vi "Test for OOB Services.vi"(8 "error in":errorcluster, 11 "address":string) -> (0 "error out":errorcluster, 3 "Found OOB Server":bool)   [LabVIEW 2026]
uses:
  Ref/reflection_client/RPC Messages/grpc_reflection_v1alpha_ServiceResponse.ctl
  Ref/reflection_client/RPC Messages/grpc_reflection_v1alpha_ServerReflectionRequest.ctl
  Ref/reflection_client/RPC Messages/grpc_reflection_v1alpha_ServerReflectionRequest_message_request/grpc_reflection_v1alpha_ServerReflectionRequest_message_request.lvclass
  Ref/reflection_client/RPC Messages/grpc_reflection_v1alpha_ServerReflectionRequest_message_request/grpc_reflection_v1alpha_ServerReflectionRequest_message_request.lvclass/grpc_reflection_v1alpha_ServerReflectionRequest_message_request.ctl
  Ref/reflection_client/RPC Messages/grpc_reflection_v1alpha_ServerReflectionResponse_message_response/grpc_reflection_v1alpha_ServerReflectionResponse_message_response.lvclass/grpc_reflection_v1alpha_ServerReflectionResponse_message_response.ctl
  Ref/reflection_client.lvlib
  Ref/reflection_client/RPC Messages/grpc_reflection_v1alpha_ServerReflectionResponse_message_response/grpc_reflection_v1alpha_ServerReflectionResponse_message_response.lvclass
panel:
  out "service":T1[](array[typedef])
  out "Success":bool
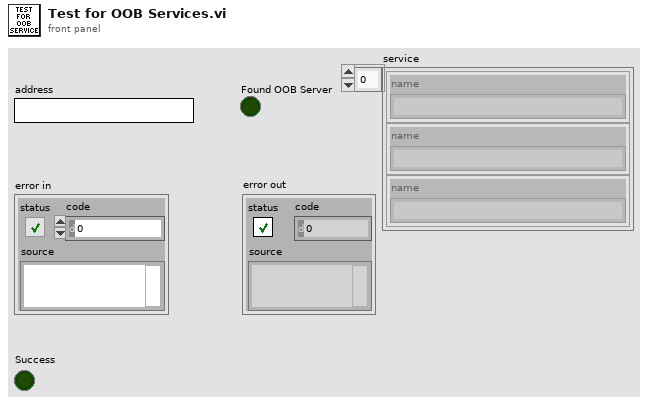
[diagram p1: front panel]
types:
  T1 = typedef "reflection_client.lvlib/grpc_reflection_v1alpha_ServiceResponse.ctl" = cluster{"name":string}
  T2 = typedef "reflection_client.lvlib/grpc_reflection_v1alpha_ServerReflectionRequest.ctl" = cluster{"host":string, "grpc_reflection_v1alpha_ServerReflectionRequest_message_request":refnum<class "grpc_reflection_v1alpha_ServerReflectionRequest_message_request.lvclass">}
  T3 = typedef "grpc-lvsupport-release.lvlib/grpcId.ctl" = u64
  T4 = typedef "reflection_client.lvlib/grpc_reflection_v1alpha_ServerReflectionResponse.ctl" = cluster{"valid_host":string, "original_request":T2, "grpc_reflection_v1alpha_ServerReflectionResponse_message_response":refnum<class "grpc_reflection_v1alpha_ServerReflectionResponse_message_response.lvclass">}
  T5 = typedef "reflection_client.lvlib/grpc_reflection_v1alpha_ListServiceResponse.ctl" = cluster{"service":T1[]}
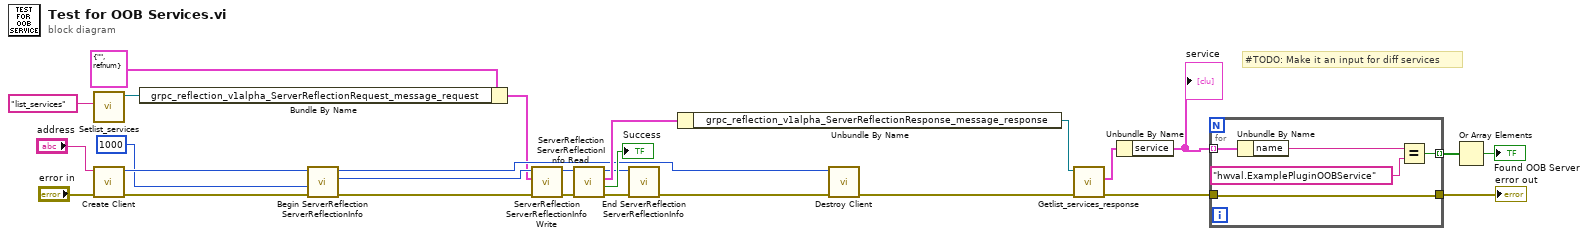
[diagram p0: block diagram]
diagram:
  # "#TODO: Make it an input for diff services"
  n1 = call "Setlist_services.vi"("Set_Val"="list_services") -> ("OneOfTemplate out"=w14:refnum<class "grpc_reflection_v1alpha_ServerReflectionRequest_message_request.lvclass">)  [unwired: 9 in, 1 out]
  n2 = call "Create Client.vi"("error in"="error in", "address"="address") -> ("error out"=w24:errorcluster, "gRPC ID Out"=w25:T3)  [unwired: 8 in]
  n3 = Bundle By Name(cluster=T2 {"host"="", "grpc_reflection_v1alpha_ServerReflectionRequest_message_request"=refnum} ("Request Data"), "grpc_reflection_v1alpha_ServerReflectionRequest_message_request"=w14) -> (w10:T2)
  n4 = call "Begin ServerReflection ServerReflectionInfo.vi"("error in"=w24, "timeout (ms)"=1000, "gRPC ID"=w25) -> ("error out"=w17:errorcluster, "Call Id Out"=w18:T3, "gRPC ID out"=w12:T3)  [unwired: 6 in]
  n5 = call "ServerReflection ServerReflectionInfo Write.vi"("error in"=w17, "Request Data"=w10, "Call ID in"=w18) -> ("error out"=w15:errorcluster, "Call ID"=w16:T3)  [unwired: 6 in, 1 out]
  n6 = call "ServerReflection ServerReflectionInfo Read.vi"("error in"=w15, "Call ID in"=w16) -> ("error out"=w9:errorcluster, "Success"=→"Success":bool, "Response Data"=w21:T4, "Call ID"=w7:T3)  [unwired: 6 in]
  n7 = call "End ServerReflection ServerReflectionInfo.vi"("error in"=w9, "Call ID in"=w7) -> ("error out"=w8:errorcluster)  [unwired: 8 in, 1 out]
  n8 = Unbundle By Name(w21) -> ("grpc_reflection_v1alpha_ServerReflectionResponse_message_response"=w20:refnum<class "grpc_reflection_v1alpha_ServerReflectionResponse_message_response.lvclass">)
  n9 = call "Destroy Client.vi"("error in"=w8, "gRPC ID"=w12) -> ("error out"=w19:errorcluster)  [unwired: 9 in]
  n10 = call "Getlist_services_response.vi"("error in (no error)"=w19, "OneOfTemplate in"=w20) -> ("error out"=w2:errorcluster, "Get_Val"=w6:T5)  [unwired: 7 in, 1 out]
  n11 = Unbundle By Name(w6) -> ("service"=w5:T1[])
  "service" <- w5
  n12 = for {
    tunnel: w5 -> [w32] mode=indexing
    tunnel: [w29] -> w4 mode=indexing
    tunnel: w2 -> [w28]
    tunnel: [w28] -> w1
    n13 = Unbundle By Name(w32) -> ("name"=w31:string)
    n14 = Equal?(x=w31, y="hwval.ExamplePluginOOBService") -> (x = y?=w29:bool)
  }
  "error out" <- w1
  n15 = Or Array Elements(Boolean array=w4) -> (logical OR=→"Found OOB Server":bool)
